vi "slopes file test.vi"() -> ()   [LabVIEW 2016]
uses:
  <vilib>/Utility/file.llb/Read Delimited Spreadsheet (DBL).vi
panel:
  out "error out":errorcluster
  out "file or folder exists?":bool
  out "all rows":dbl[][](array[numeric])
  in  "error in (no error)":errorcluster
  in  "Slopes File Path":path=path "C:/Cascade/Data/Output Files/slopes.csv"
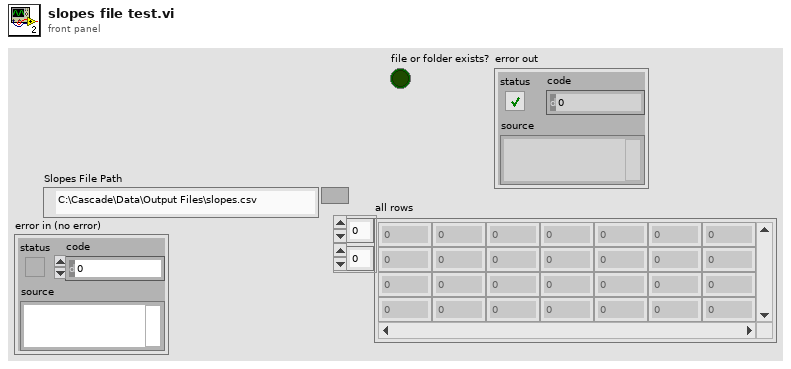
[diagram p1: front panel]
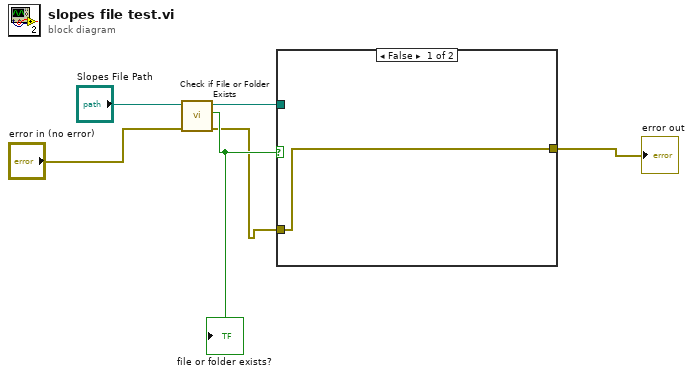
[diagram p0: block diagram]
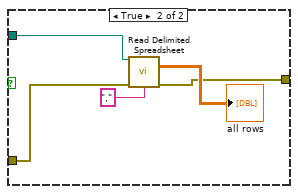
[diagram p2: hidden frame]
diagram:
  n1 = call <vilib>:"Check if File or Folder Exists.vi"("error in (no error)"="error in (no error)", "path"="Slopes File Path") -> ("error out"=w3:errorcluster, "file or folder exists?"=w4:bool, "dup path"=w2:path)  [unwired: 7 in]
  "file or folder exists?" <- w4
  n2 = case shown="False" w4 {
    tunnel: w3 -> [w7 w11]
    tunnel: w2 -> [_ w12]
    tunnel: [w7 w8] -> w1
    frame False {
    }
    frame True {
      n3 = call-poly <vilib>:"Read Delimited Spreadsheet.vi"("file path (dialog if empty)"=w12, "error in (no error)"=w11, "delimiter (\\t)"="," ("delimiter (\\t)")) -> ("all rows"=→"all rows":dbl[][], "error out"=w8:errorcluster)  [unwired: 7 in, 4 out]
    }
  }
  "error out" <- w1
